vi "FTA10-1000Control_1.vi"(0 "Port":string="ª\u0001&\u0000'", 1 "baud rate (9600)":u32=9600 caption="波特率(9600)", 2 "function":u16(ring) items=["Open", "SetVolt", "SetCurrent", "SetVoltAndCurrent", "ReadVoltAndCurrent", "OutPut ON", "OutPUt OFF", "Close"], 3 "volt set (V)":u32, 4 "curr set (MA)":dbl) -> (20 "volt out":dbl, 21 "curr out":dbl, 22 "result":i32=2)   [LabVIEW 2013]
uses:
  <vilib>/Instr/_visa.llb/VISA Configure Serial Port (Instr).vi
panel:
  out "读取缓冲区 2":string
  out "返回数":u32
  out "读取缓冲区":string
  out "Out":string
  out "error out":errorcluster
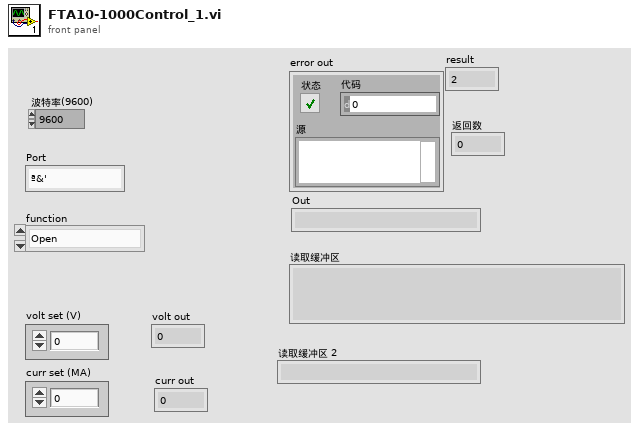
[diagram p1: front panel]
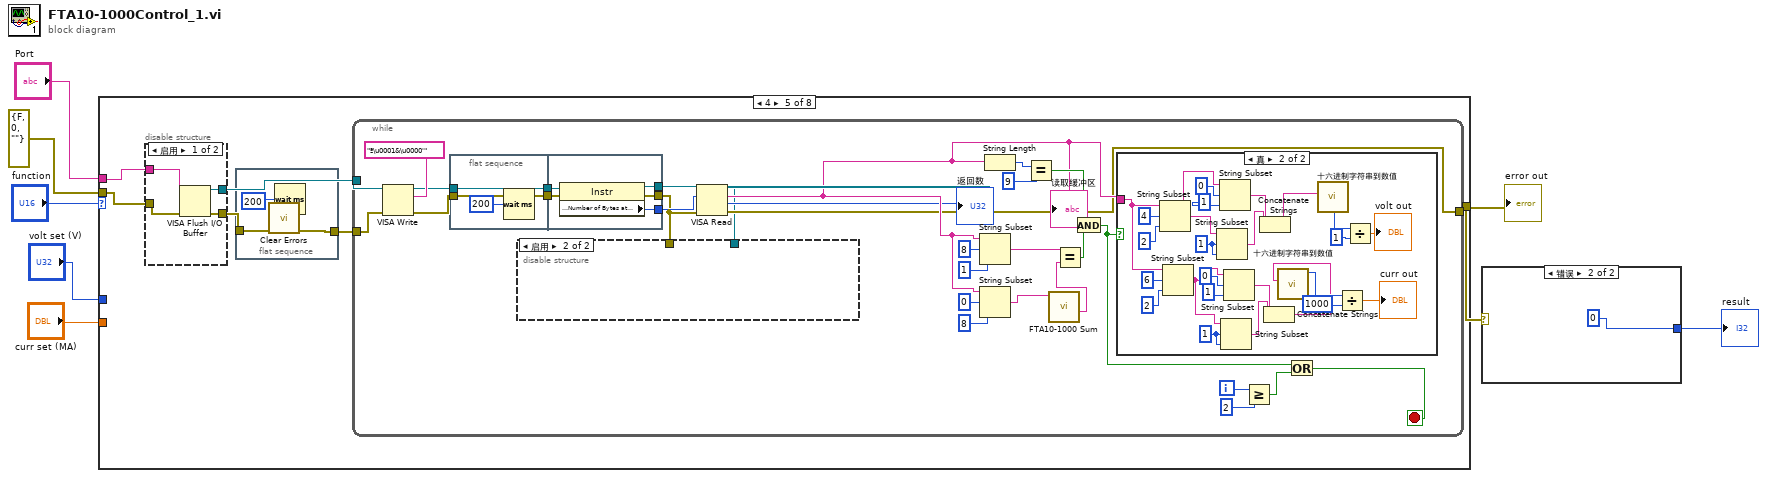
[diagram p0: block diagram]
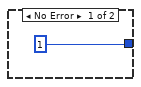
[diagram p2: hidden frame]
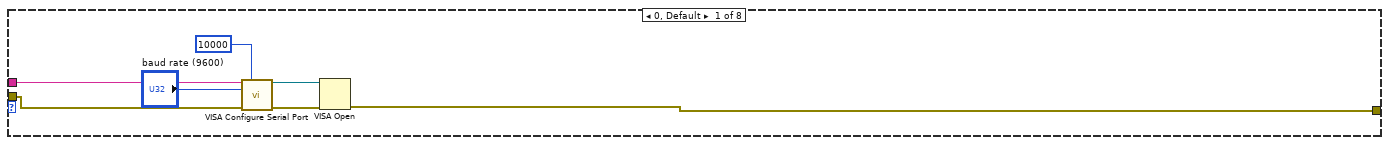
[diagram p3: hidden frame]
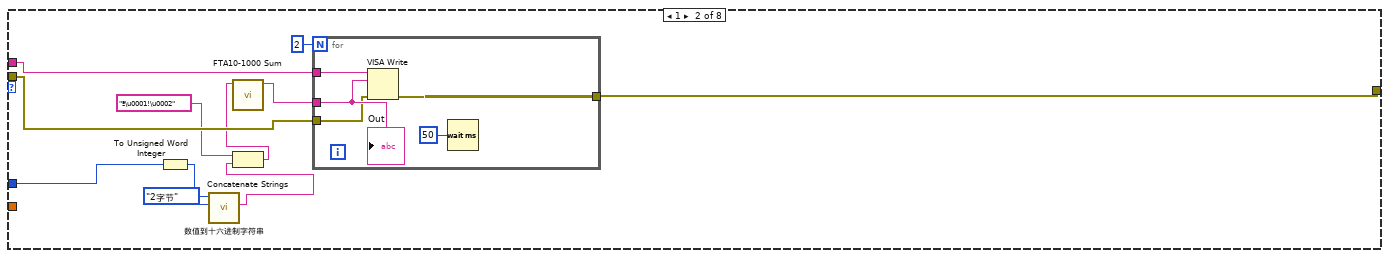
[diagram p4: hidden frame]
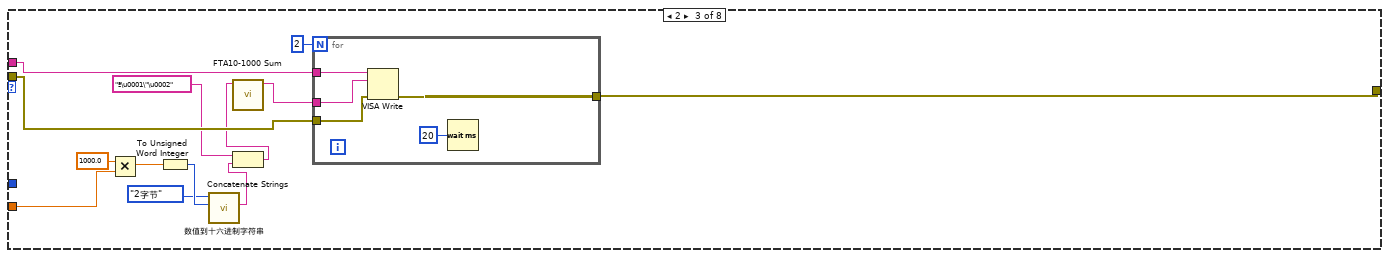
[diagram p5: hidden frame]
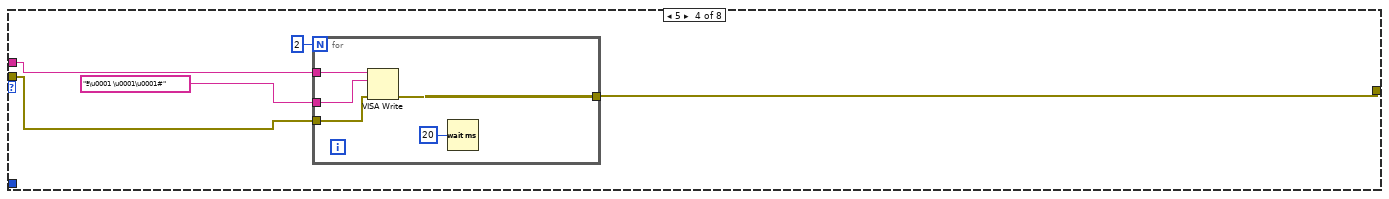
[diagram p6: hidden frame]
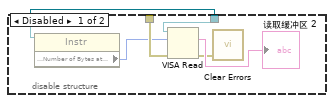
[diagram p8: hidden frame]
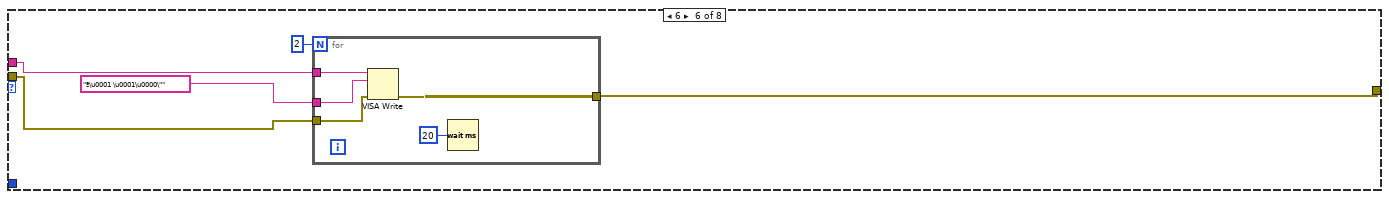
[diagram p10: hidden frame]
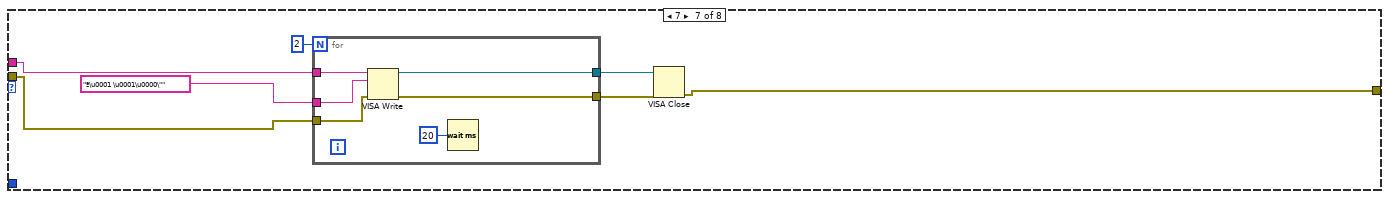
[diagram p11: hidden frame]
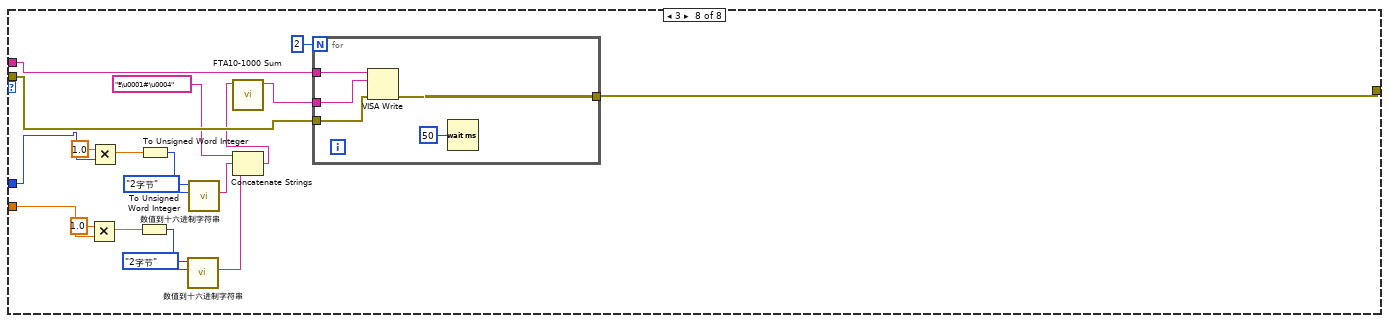
[diagram p12: hidden frame]
diagram:
  n1 = case shown="4" "function" {
    tunnel: "Port" -> [w12 w23 w41 w52 w62 w145 w157 w181]
    tunnel: errorcluster {"status"=FALSE, "code"=0, "source"=""} ("error in (no error)") -> [w11 w22 w40 w51 w61 w144 w156 w180]
    tunnel: [w10 w21 w39 w50 w64 w143 w152 w179] -> w2
    tunnel: "curr set (MA)" -> [_ _ w32 _ _ _ _ w172]
    tunnel: "volt set (V)" -> [_ w15 _ _ _ _ _ w167]
    frame 0, Default {
      n2 = call-poly "VISA Configure Serial Port"("VISA resource name"=w12, "timeout (10sec)"=u32 10000, "baud rate (9600)"="baud rate (9600)", "error in (no error)"=w11) -> ("VISA resource name out"=w14:refnum<visa-resource-name>, "error out"=w13:errorcluster)  [unwired: 10 in]
      n3 = VISA Open(error in (no error)=w13, VISA resource name=w14) -> (error out=w10:errorcluster)  [unwired: 3 in, 1 out]
    }
    frame 1 {
      n4 = To Unsigned Word Integer(number=w15) -> (unsigned 16bit integer=w20:u16)
      n5 = call "数值到十六进制字符串.vi"("Numeric"=w20, "转换字节数"=enum16{"1字节", "2字节", "4字节", "3字节"}."2字节") -> ("二字节互换"=w16:string)  [unwired: 8 in, 1 out]
      n6 = Concatenate Strings("ª\u0001!\u0002" ("In"), w16) -> (w17:string)
      n7 = call "FTA10-1000 Sum.vi"("In"=w17) -> ("Out"=w25:string)  [unwired: 8 in, 2 out]
      n8 = for {
        N: 2 -> [_]
        tunnel: [w30] -> w21
        tunnel: w23 -> [w29]
        tunnel: w25 -> [w28]
        tunnel: w22 -> [w27]
        n9 = VISA Write(VISA resource name=w29, write buffer=w28, error in (no error)=w27) -> (error out=w30:errorcluster)  [unwired: 2 out]
        n10 = Wait (ms)(milliseconds to wait=u32 50 ("等待时间（毫秒）")) -> ()  [unwired: 1 out]
        "Out" <- w28
      }
    }
    frame 2 {
      n11 = Multiply(x=1000.0, y=w32) -> (x*y=w38:dbl)
      n12 = To Unsigned Word Integer(number=w38) -> (unsigned 16bit integer=w36:u16)
      n13 = call "数值到十六进制字符串.vi"("Numeric"=w36, "转换字节数"=enum16{"1字节", "2字节", "4字节", "3字节"}."2字节") -> ("二字节互换"=w31:string)  [unwired: 8 in, 1 out]
      n14 = Concatenate Strings("ª\u0001\"\u0002" ("In"), w31) -> (w33:string)
      n15 = call "FTA10-1000 Sum.vi"("In"=w33) -> ("Out"=w43:string)  [unwired: 8 in, 2 out]
      n16 = for {
        N: 2 -> [_]
        tunnel: [w48] -> w39
        tunnel: w41 -> [w47]
        tunnel: w43 -> [w46]
        tunnel: w40 -> [w45]
        n17 = VISA Write(VISA resource name=w47, write buffer=w46, error in (no error)=w45) -> (error out=w48:errorcluster)  [unwired: 2 out]
        n18 = Wait (ms)(milliseconds to wait=u32 20 ("等待时间（毫秒）")) -> ()  [unwired: 1 out]
      }
    }
    frame 5 {
      n19 = for {
        N: 2 -> [_]
        tunnel: [w58] -> w50
        tunnel: w52 -> [w57]
        tunnel: "ª\u0001 \u0001\u0001#" ("In") -> [w56]
        tunnel: w51 -> [w55]
        n20 = VISA Write(VISA resource name=w57, write buffer=w56, error in (no error)=w55) -> (error out=w58:errorcluster)  [unwired: 2 out]
        n21 = Wait (ms)(milliseconds to wait=u32 20 ("等待时间（毫秒）")) -> ()  [unwired: 1 out]
      }
    }
    frame 4 {
      n22 = disable-structure shown="启用" {
        disable-tunnel: w62 -> [w68 w70]
        disable-tunnel: w61 -> [w67 w69]
        disable-tunnel: [w66 w70] -> w60
        disable-tunnel: [w65 w69] -> w59
        frame Enabled {
          n23 = VISA Flush I/O Buffer(VISA resource name=w68, error in (no error)=w67) -> (VISA resource name out=w66:refnum<visa-resource-name>, error out=w65:errorcluster)  [unwired: 1 in]
        }
        frame Disabled {
        }
      }
      n24 = flat-sequence {
        tunnel: [w73] -> w63
        tunnel: w59 -> [w72]
        frame #0 {
          n25 = call <vilib>:"Clear Errors.vi"("error in (no error)"=w72) -> ("error out"=w73:errorcluster)  [unwired: 6 in]
          n26 = Wait (ms)(milliseconds to wait=u32 200 ("等待时间（毫秒）")) -> ()  [unwired: 1 out]
        }
      }
      n27 = while {
        tunnel: [w82] -> w64
        tunnel: w60 -> [w102]
        tunnel: w63 -> [w83]
        i -> [w85]
        stop <- w77 stop-if-true
        n28 = VISA Write(VISA resource name=w102, write buffer="ª\u0001&\u0000'" ("In"), error in (no error)=w83) -> (VISA resource name out=w100:refnum<visa-resource-name>, error out=w87:errorcluster)  [unwired: 1 out]
        n29 = flat-sequence {
          tunnel: w87 -> [w110]
          tunnel: w100 -> [w111]
          tunnel: [w111] -> w81
          tunnel: [w110] -> w80
          tunnel: [w116] -> w101
          tunnel: [w114] -> w88
          tunnel: [w112] -> w75
          tunnel: w81 -> [w115]
          tunnel: w80 -> [w113]
          frame #0 {
            n30 = Wait (ms)(milliseconds to wait=u32 200 ("等待时间（毫秒）")) -> ()  [unwired: 1 out]
          }
          frame #1 {
            n31 = property class="Instr"(reference=w115, error in=w113) -> (reference out=w114:refnum<visa-resource-name>, error out=w112:errorcluster, "Serial Settings:Number of Bytes at Serial Port"=w116:u32)
          }
        }
        n32 = VISA Read(VISA resource name=w88, byte count=w101, error in (no error)=w75) -> (VISA resource name out=w74:refnum<visa-resource-name>, read buffer=w86:string, return count=→"返回数":u32, error out=w82:errorcluster)
        "读取缓冲区" <- w86
        n33 = disable-structure shown="启用" {
          disable-tunnel: w75 -> [w107 _]
          disable-tunnel: w74 -> [w105 _]
          frame Disabled {
            n34 = property class="Instr"(reference=w105) -> ("Serial Settings:Number of Bytes at Serial Port"=w106:u32)  [unwired: 1 in, 2 out]
            n35 = VISA Read(VISA resource name=w105, byte count=w106, error in (no error)=w107) -> (read buffer=→"读取缓冲区 2":string, error out=w104:errorcluster)  [unwired: 2 out]
            n36 = call <vilib>:"Clear Errors.vi"("error in (no error)"=w104) -> ()  [unwired: 6 in, 1 out]
          }
          frame Enabled {
          }
        }
        n37 = String Subset(string=w86, offset (0)=8 ("偏移量(0)"), length (rest)=1 ("长度（剩余）")) -> (substring=w92:string)
        n38 = String Subset(string=w86, offset (0)=0 ("偏移量(0)"), length (rest)=8 ("长度（剩余）")) -> (substring=w93:string)
        n39 = String Length(string=w86) -> (length=w99:i32)
        n40 = Equal?(x=w99, y=9) -> (x = y?=w90:bool)
        n41 = call "FTA10-1000 Sum.vi"("In"=w93) -> ("Lsum_String"=w91:string)  [unwired: 8 in, 2 out]
        n42 = Equal?(x=w92, y=w91) -> (x = y?=w89:bool)
        n43 = And(x=w90, y=w89) -> (x .and. y?=w79:bool)
        n44 = case shown="真" w79 {
          tunnel: w86 -> [_ w131]
          frame False {
          }
          frame True {
            w121 = 1 ("偏移量(0)")
            w127 = 1 ("偏移量(0)")
            n45 = String Subset(string=w131, offset (0)=4 ("偏移量(0)"), length (rest)=2 ("长度（剩余）")) -> (substring=w128:string)
            n46 = String Subset(string=w131, offset (0)=6 ("偏移量(0)"), length (rest)=2 ("长度（剩余）")) -> (substring=w117:string)
            n47 = String Subset(string=w128, offset (0)=w127, length (rest)=w127) -> (substring=w124:string)
            n48 = String Subset(string=w128, offset (0)=0 ("长度（剩余）"), length (rest)=1 ("长度（剩余）")) -> (substring=w125:string)
            n49 = String Subset(string=w117, offset (0)=w121, length (rest)=w121) -> (substring=w123:string)
            n50 = String Subset(string=w117, offset (0)=0 ("长度（剩余）"), length (rest)=1 ("长度（剩余）")) -> (substring=w122:string)
            n51 = Concatenate Strings(w124, w125) -> (w126:string)
            n52 = Concatenate Strings(w123, w122) -> (w118:string)
            n53 = call "十六进制字符串到数值.vi"("字符串"=w118) -> ("数值"=w134:i32)  [unwired: 9 in, 1 out]
            n54 = call "十六进制字符串到数值.vi"("字符串"=w126) -> ("数值"=w139:i32)  [unwired: 9 in, 1 out]
            n55 = Divide(x=w134, y=1000) -> (x/y=→"curr out":dbl)
            n56 = Divide(x=w139, y=1) -> (x/y=→"volt out":dbl)
          }
        }
        n57 = Greater Or Equal?(x=w85, y=2) -> (x >= y?=w78:bool)
        n58 = Or(x=w79, y=w78) -> (x .or. y?=w77:bool)
      }
    }
    frame 6 {
      n59 = for {
        N: 2 -> [_]
        tunnel: [w151] -> w143
        tunnel: w145 -> [w150]
        tunnel: "ª\u0001 \u0001\u0000\"" ("In") -> [w149]
        tunnel: w144 -> [w148]
        n60 = VISA Write(VISA resource name=w150, write buffer=w149, error in (no error)=w148) -> (error out=w151:errorcluster)  [unwired: 2 out]
        n61 = Wait (ms)(milliseconds to wait=u32 20 ("等待时间（毫秒）")) -> ()  [unwired: 1 out]
      }
    }
    frame 7 {
      n62 = for {
        N: 2 -> [_]
        tunnel: [w164] -> w153
        tunnel: w157 -> [w163]
        tunnel: "ª\u0001 \u0001\u0000\"" ("In") -> [w162]
        tunnel: w156 -> [w161]
        tunnel: [w159] -> w154
        n63 = VISA Write(VISA resource name=w163, write buffer=w162, error in (no error)=w161) -> (VISA resource name out=w159:refnum<visa-resource-name>, error out=w164:errorcluster)  [unwired: 1 out]
        n64 = Wait (ms)(milliseconds to wait=u32 20 ("等待时间（毫秒）")) -> ()  [unwired: 1 out]
      }
      n65 = VISA Close(VISA resource name=w154, error in (no error)=w153) -> (error out=w152:errorcluster)
    }
    frame 3 {
      n66 = Multiply(x=1.0, y=w172) -> (x*y=w178:dbl)
      n67 = Multiply(x=1.0, y=w167) -> (x*y=w168:dbl)
      n68 = To Unsigned Word Integer(number=w178) -> (unsigned 16bit integer=w176:u16)
      n69 = To Unsigned Word Integer(number=w168) -> (unsigned 16bit integer=w170:u16)
      n70 = call "数值到十六进制字符串.vi"("Numeric"=w176, "转换字节数"=enum16{"1字节", "2字节", "4字节", "3字节"}."2字节") -> ("二字节互换"=w165:string)  [unwired: 8 in, 1 out]
      n71 = call "数值到十六进制字符串.vi"("Numeric"=w170, "转换字节数"=enum16{"1字节", "2字节", "4字节", "3字节"}."2字节") -> ("二字节互换"=w166:string)  [unwired: 8 in, 1 out]
      n72 = Concatenate Strings("ª\u0001#\u0004" ("In"), w166, w165) -> (w173:string)
      n73 = call "FTA10-1000 Sum.vi"("In"=w173) -> ("Out"=w183:string)  [unwired: 8 in, 2 out]
      n74 = for {
        N: 2 -> [_]
        tunnel: [w188] -> w179
        tunnel: w181 -> [w187]
        tunnel: w183 -> [w186]
        tunnel: w180 -> [w185]
        n75 = VISA Write(VISA resource name=w187, write buffer=w186, error in (no error)=w185) -> (error out=w188:errorcluster)  [unwired: 2 out]
        n76 = Wait (ms)(milliseconds to wait=u32 50 ("等待时间（毫秒）")) -> ()  [unwired: 1 out]
      }
    }
  }
  "error out" <- w2
  n77 = case shown="错误" w2 {
    tunnel: [1 ("y") 0 ("y")] -> w1
    frame No Error {
    }
    frame Error {
    }
  }
  "result" <- w1
